vi "New Drive Train Status.vi"(8 "error in (no error)":errorcluster, 10 "Drive Train Status":T1 {"Right Power Setpoint" min=-1.0 max=1.0 step=0.1 scale=-1.0..1.0; "Left Power Setpoint" min=-1.0 max=1.0 step=0.1 scale=-1.0..1.0; "Right Power" min=-1.0 max=1.0 step=0.1 scale=-1.0..1.0; "Left Power" min=-1.0 max=1.0 step=0.1 scale=-1.0..1.0}, 11 "Drive Train Command in":refnum<class "Drive Train Command.lvclass">) -> (0 "error out":errorcluster, 3 "Drive Train Command out":refnum<class "Drive Train Command.lvclass">)   [LabVIEW 2014, in "Logical Systems.lvlib" / "Drive Train.lvlib" / "Drive Train Command.lvlib" / "Drive Train Command.lvclass"]
uses:
  Drive Train Command.lvclass
  Drive Train Class/Drive Train Status.ctl
  <vilib>/ActorFramework/Actor/Actor.lvclass/Actor.ctl
  <vilib>/ActorFramework/Actor/Actor.lvclass
  Drive Train Messages/Set Power Msg/Set Power Msg.lvclass
  Drive Train Class/Drive Train.lvclass
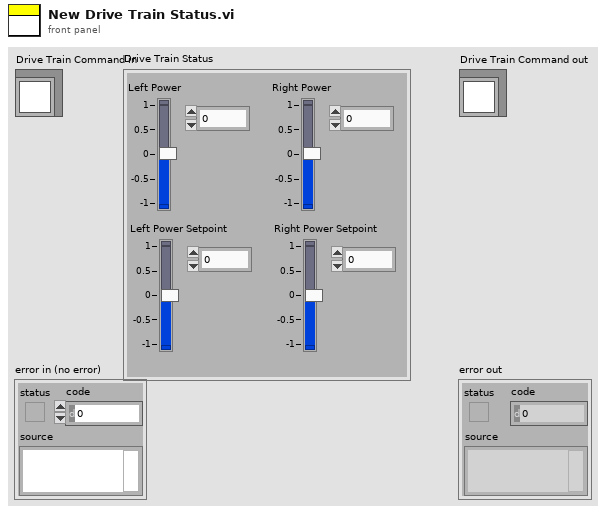
[diagram p1: front panel]
types:
  T1 = typedef "Logical Systems.lvlib/Drive Train.lvlib/Drive Train.lvclass/Drive Train Status.ctl" = cluster{"Left Power":dbl, "Right Power":dbl, "Left Power Setpoint":dbl, "Right Power Setpoint":dbl}
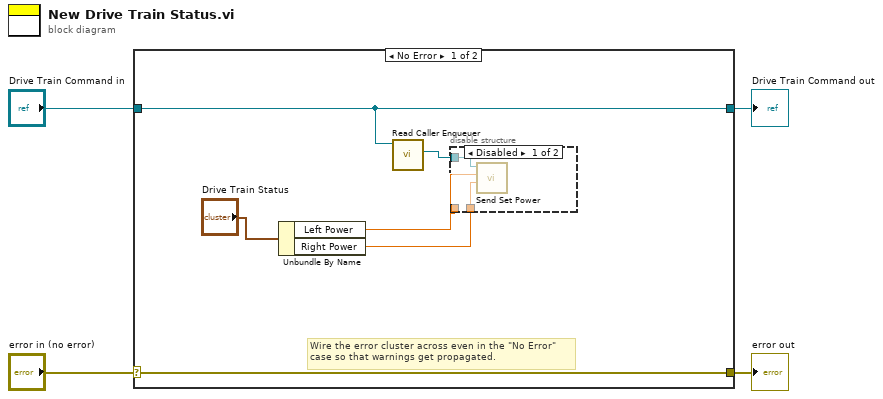
[diagram p0: block diagram]
diagram:
  n1 = case shown="No Error" "error in (no error)" {
    selector: "error in (no error)" -> [w10 w15]
    tunnel: [w10 w15] -> w3
    tunnel: [w9 w14] -> w1
    tunnel: "Drive Train Command in" -> [w9 w14]
    frame No Error {
      # "Wire the error cluster across even in the \"No Error\"\ncase so that warnings get propagated."
      n2 = Unbundle By Name("Drive Train Status") -> ("Left Power"=w6:dbl, "Right Power"=w5:dbl)
      n3 = call <vilib>:"Read Caller Enqueuer.vi"("Actor"=w9) -> ("Caller Enqueuer"=w8:refnum<class "Message Enqueuer.lvclass">)  [unwired: 10 in]
      n4 = disable-structure shown="Disabled" {
        disable-tunnel: w8 -> [w13 _]
        disable-tunnel: w6 -> [w12 _]
        disable-tunnel: w5 -> [w11 _]
        frame Disabled {
          n5 = call "Send Set Power.vi"("Right Power"=w11, "Left Power"=w12, "Message Enqueuer"=w13) -> ()  [unwired: 7 in, 2 out]
        }
        frame Enabled {
        }
      }
    }
    frame Error {
    }
  }
  "error out" <- w3
  "Drive Train Command out" <- w1
